vi "Test_InsertRemoveCount.vi"(8 "error in (no error)":errorcluster, 11 "TestCase in":refnum<class "BufferedArray_Functional.lvclass">) -> (0 "error out":errorcluster, 3 "TestCase out":refnum<class "BufferedArray_Functional.lvclass">)   [LabVIEW 2009, in "BufferedArray_Functional.lvclass"]
uses:
  BufferedArray_Functional.lvclass
  BufferedArray_Functional.lvclass/BufferedArray_Functional.ctl
  source/Lists/List/List.lvclass
  source/Lists.Interfaces/String/String.lvclass
  UnitTestComparisons/UnitTestComparisons.lvlib
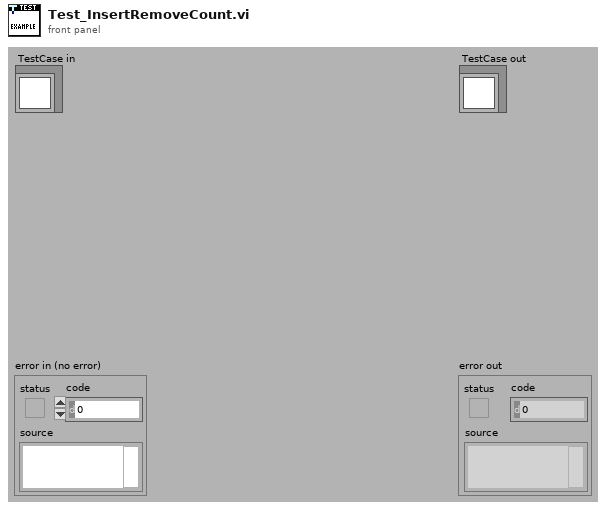
[diagram p1: front panel]
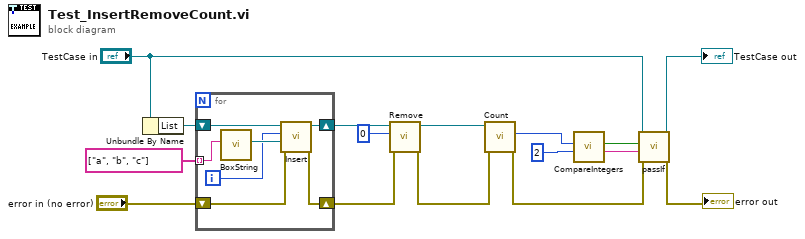
[diagram p0: block diagram]
diagram:
  n1 = Unbundle By Name("TestCase in") -> ("List"=w12:refnum<class "List.lvclass">)
  n2 = for {
    tunnel: string[] ["a", "b", "c"] -> [w20] mode=indexing
    shift-right: [w22] -> w9
    shift-left: w12 -> [w23]
    shift-right: [w17] -> w6
    shift-left: "error in (no error)" -> [w18]
    i -> [w19]
    n3 = call "BoxString.vi"("String"=w20) -> ("String out"=w21:refnum<class "String.lvclass">)  [unwired: 10 in]
    n4 = call-dynamic "Insert.vi"("error in (no error)"=w18, "Item"=w21, "Index"=w19, "List in"=w23) -> ("error out"=w17:errorcluster, "List out"=w22:refnum<class "List.lvclass">)  [unwired: 6 in]
  }
  n5 = call-dynamic "Remove.vi"("error in (no error)"=w6, "Index"=0, "List in"=w9) -> ("error out"=w5:errorcluster, "List out"=w8:refnum<class "List.lvclass">)  [unwired: 6 in, 1 out]
  n6 = call-dynamic "Count.vi"("error in (no error)"=w5, "List in"=w8) -> ("error out"=w13:errorcluster, "Number of Items"=w4:i32)  [unwired: 7 in, 1 out]
  n7 = call "CompareIntegers.vi"("Expected Value"=2 ("x"), "Actual Value"=w4) -> ("Message"=w2:string, "Equal?"=w1:bool)  [unwired: 8 in]
  n8 = call-dynamic "passIf.vi"("error in (no error)"=w13, "message (\"\")"=w2, "pass"=w1, "TestCase in"="TestCase in") -> ("error out"=→"error out":errorcluster, "TestCase out"=→"TestCase out":refnum<class "BufferedArray_Functional.lvclass">)  [unwired: 6 in]
